vi "Control-con-Mouse-final.vi"() -> ()   [LabVIEW 2024]
uses:
  <vilib>/Utility/inputDevices.llb/mouseAcquire.vi
  <vilib>/Utility/inputDevices.llb/closeMouse.vi
panel:
  out "Dioptrias Finales":dbl
  out "Vertical":i32
  in  "stop":bool
  out "axis info":T1
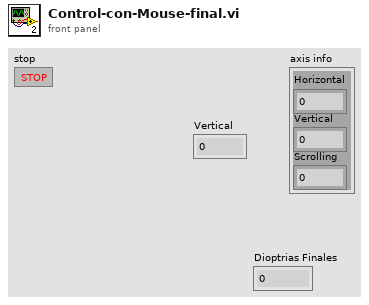
[diagram p1: front panel]
types:
  T1 = cluster{"Horizontal":i32, "Vertical":i32, "Scrolling":i32}
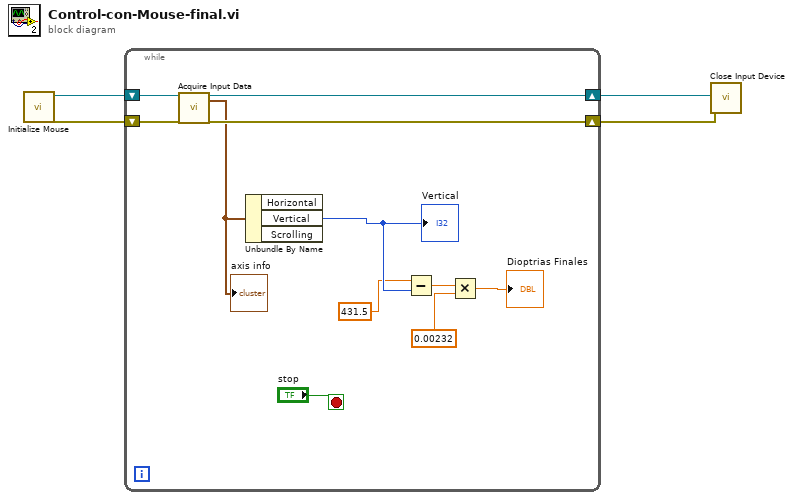
[diagram p0: block diagram]
diagram:
  n1 = call <vilib>:"Initialize Mouse.vi"() -> ("error out"=w2:errorcluster, "device ID"=w4:refnum<k1>)  [unwired: 10 in]
  n2 = while {
    shift-right: [w14] -> w3
    shift-left: w4 -> [w15]
    shift-right: [w12] -> w1
    shift-left: w2 -> [w13]
    stop <- "stop" stop-if-true
    n3 = call-poly <vilib>:"Acquire Input Data.vi"("device ID"=w15, "error in (no error)"=w13) -> ("device ID"=w14:refnum<k1>, "axis info"=w10:T1, "error out"=w12:errorcluster)  [unwired: 14 in, 1 out]
    "axis info" <- w10
    n4 = Unbundle By Name(w10) -> ("Vertical"=w9:i32)  [unwired: 2 out]
    "Vertical" <- w9
    n5 = Subtract(x=431.5, y=w9) -> (x-y=w7:dbl)
    n6 = Multiply(x=w7, y=0.00232) -> (x*y=→"Dioptrias Finales":dbl)
  }
  n7 = call-poly <vilib>:"Close Input Device.vi"("error in (no error)"=w1, "device ID"=w3) -> ()  [unwired: 8 in, 1 out]
